vi "RSZVB Set Calibration Kit Label.vi"(8 "error in (no error)":errorcluster {"code" format="%.0x"}, 9 "Label":string, 10 "Calibration Kit Name":string, 11 "VISA session":refnum<visa-resource-name>) -> (0 "error out":errorcluster {"code" format="%.0x"}, 3 "dup VISA session":refnum<visa-resource-name>)   [LabVIEW 2011]
doc: "This VI assigns a label to an imported or user-defined calibration kit.\n\nRemote-control command(s):\n[SENSe<Ch>:]CORRection:CKIT:LABel '<ckit_name>', '<label>'"
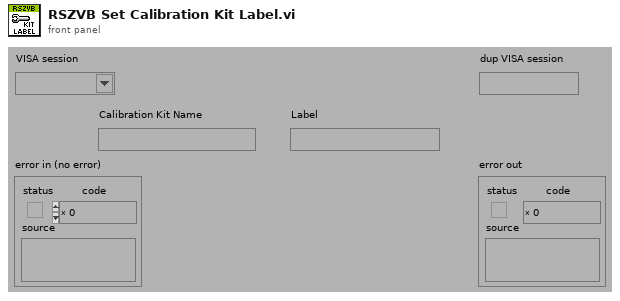
[diagram p1: front panel]
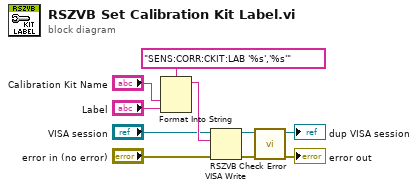
[diagram p0: block diagram]
diagram:
  n1 = Format Into String(format string="SENS:CORR:CKIT:LAB '%s','%s'", "Calibration Kit Name", "Label") -> (resulting string=w10:string)  [unwired: 2 in, 1 out]
  n2 = VISA Write(VISA resource name="VISA session", write buffer=w10, error in (no error)="error in (no error)") -> (VISA resource name out=w8:refnum<visa-resource-name>, error out=w9:errorcluster)  [unwired: 1 out]
  n3 = call "RSZVB Check Error.vi"("error in (no error)"=w9, "VISA session"=w8) -> ("error out"=→"error out":errorcluster, "dup VISA session"=→"dup VISA session":refnum<visa-resource-name>)  [unwired: 8 in]
